vi "uni-bi NRZ.vi"() -> ()   [LabVIEW 2014]
uses:
  <vilib>/Analysis/NI_AALPro.lvlib
panel:
  in  "frequency":i32
  out "bipolar NRZ":dbl[](graph)
  in  "frequency":i32
  out "unipolar NRZ":dbl[](graph)
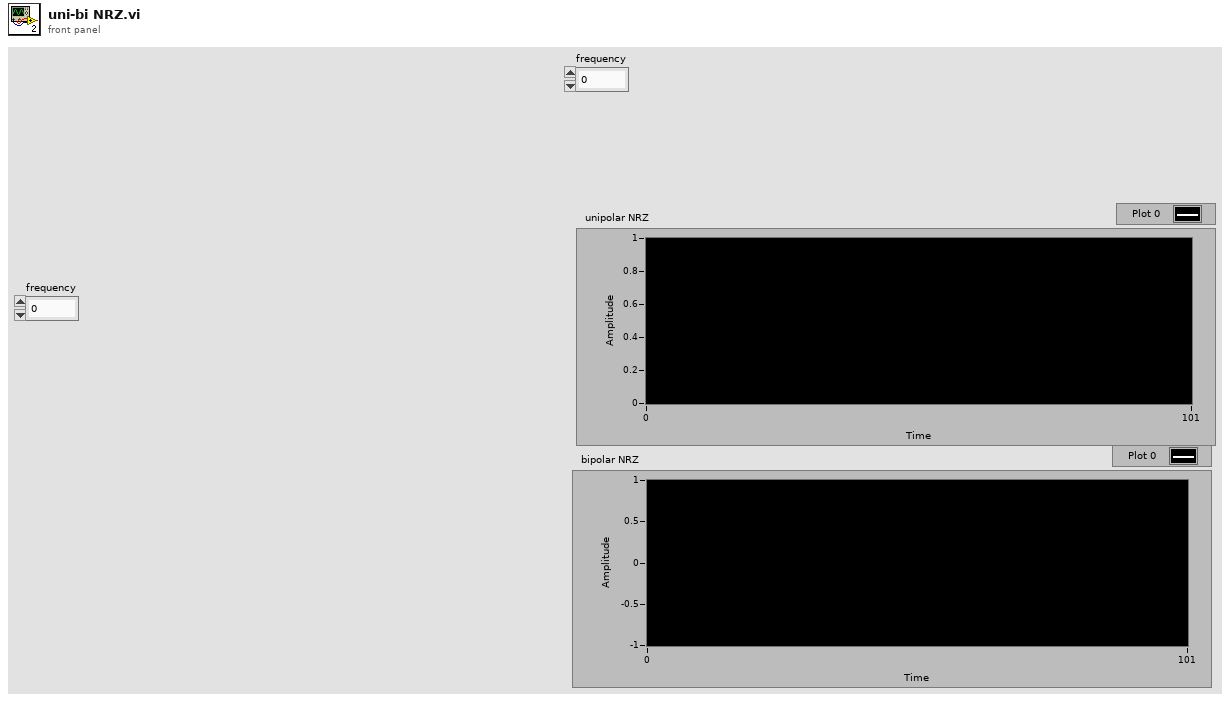
[diagram p1: front panel]
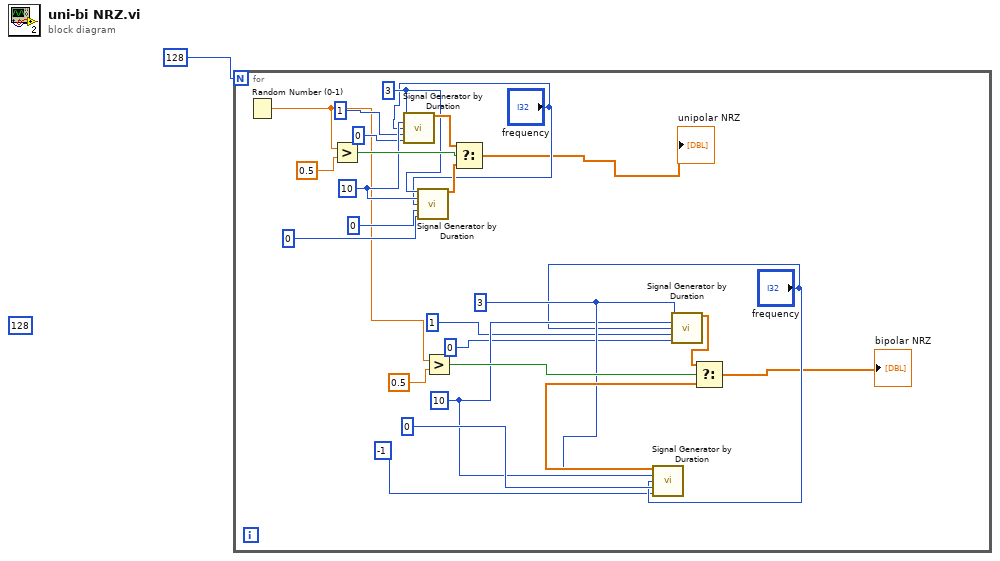
[diagram p0: block diagram]
diagram:
  (unwired) 128
  n1 = for {
    N: 128 -> [_]
    w9 = 10
    w10 = 3
    w20 = 10
    w21 = 3
    n2 = Random Number (0-1)() -> (number: 0 to 1=w6:dbl)
    n3 = Greater?(x=w6, y=0.5) -> (0:w25:bool)
    n4 = call <vilib>:"Signal Generator by Duration.vi"("signal type"=w21, "# of samples"=w20, "frequency"="frequency", "amplitude"=1, "dc offset"=0) -> ("signal"=w24:dbl[])  [unwired: 7 in, 3 out]
    n5 = call <vilib>:"Signal Generator by Duration.vi"("signal type"=w21, "# of samples"=w20, "frequency"="frequency", "amplitude"=0, "dc offset"=0) -> ("signal"=w23:dbl[])  [unwired: 7 in, 3 out]
    n6 = Greater?(x=w6, y=0.5) -> (0:w14:bool)
    n7 = Select(t=w24, s=w25, f=w23) -> (s? t:f=→"unipolar NRZ":dbl[])
    n8 = call <vilib>:"Signal Generator by Duration.vi"("signal type"=w10, "# of samples"=w9, "frequency"="frequency", "amplitude"=0, "dc offset"=-1) -> ("signal"=w12:dbl[])  [unwired: 7 in, 3 out]
    n9 = call <vilib>:"Signal Generator by Duration.vi"("signal type"=w10, "# of samples"=w9, "frequency"="frequency", "amplitude"=1, "dc offset"=0) -> ("signal"=w13:dbl[])  [unwired: 7 in, 3 out]
    n10 = Select(t=w13, s=w14, f=w12) -> (s? t:f=→"bipolar NRZ":dbl[])
  }
